vi "host.vi"() -> ()   [LabVIEW 2020]
uses:
  b4957acc-33c7-4f51-b6c8-be02e890b770.vi
  <vilib>/Array/Sort 2D Array - Pop Stack.vi
  <vilib>/Array/Sort 2D Array - Push Stack.vi
  b4957acc-33c7-4f51-b6c8-be02e890b770.vi/269d4b3b-47f5-49e3-8884-44851e4dd9d5.vi
  b4957acc-33c7-4f51-b6c8-be02e890b770.vi/6d99389c-673d-4efb-bf33-19b32bcf4cf8.vi
  <vilib>/FPGAPlugInAG/cRIO-9035/niLvFpga_Open_cRIO-9035.vi
  <vilib>/FPGAPlugInAG/cRIO-9035/niLvFpga_Reset_cRIO-9035.vi
  <vilib>/Utility/error.llb/Error Cluster From Error Code.vi
  <vilib>/rvi/errors/niLvFpgaAdjustHostInterfaceError.vi
  <vilib>/FPGAPlugInAG/cRIO-9035/niLvFpga_Run_cRIO-9035.vi
  <vilib>/FPGAPlugInAG/cRIO-9035/niLvFpga_Close_cRIO-9035.vi
  <vilib>/rvi/interface/nirviOpenFPGA/nirviOpenFPGA.xnode
  FPGA Bitfiles/project_FPGATarget_target_0bYJLxOeBdk.lvbitx
  target.vi
  <vilib>/rvi/interface/nirviMethod/nirviMethod.xnode
  <vilib>/rvi/interface/nirviReadWriteControl/nirviReadWriteControl.xnode
  <vilib>/rvi/interface/nirviCloseFPGA/nirviCloseFPGA.xnode
  <vilib>/Analysis/NI_AALBase.lvlib
  <vilib>/FPGAPlugInAG/cRIO-9035/niLvFpga_StartFifo_cRIO-9035.vi
  <vilib>/rvi/errors/niLvFpgaMergeErrorWithErrorCode.vi
  <vilib>/FPGAPlugInAG/cRIO-9035/niLvFpga_ReadFifo_cRIO-9035.vi
  <vilib>/FPGAPlugInAG/cRIO-9035/niLvFpga_WriteFifo_cRIO-9035.vi
  NiFpgaLv.dll
panel:
  out "LabVIEW sorted array with index 2":sgl[][](array[numeric])
  out "FPGA sorted array with index":sgl[][](array[numeric])
  out "Elements Remaining index":u32
  out "Data":sgl[](array[numeric])
  out "error out":errorcluster
  out "Timed Out? FIFO out IMG":bool
  out "Timed Out? FIFO out REAL":bool
  out "Timed Out? FIFO in REAL":bool
  out "input data":sgl[](graph)
  out "sort time (ms)":dbl
  out "Elements Remaining":u32
  out "Real sorted signal":sgl[](graph)
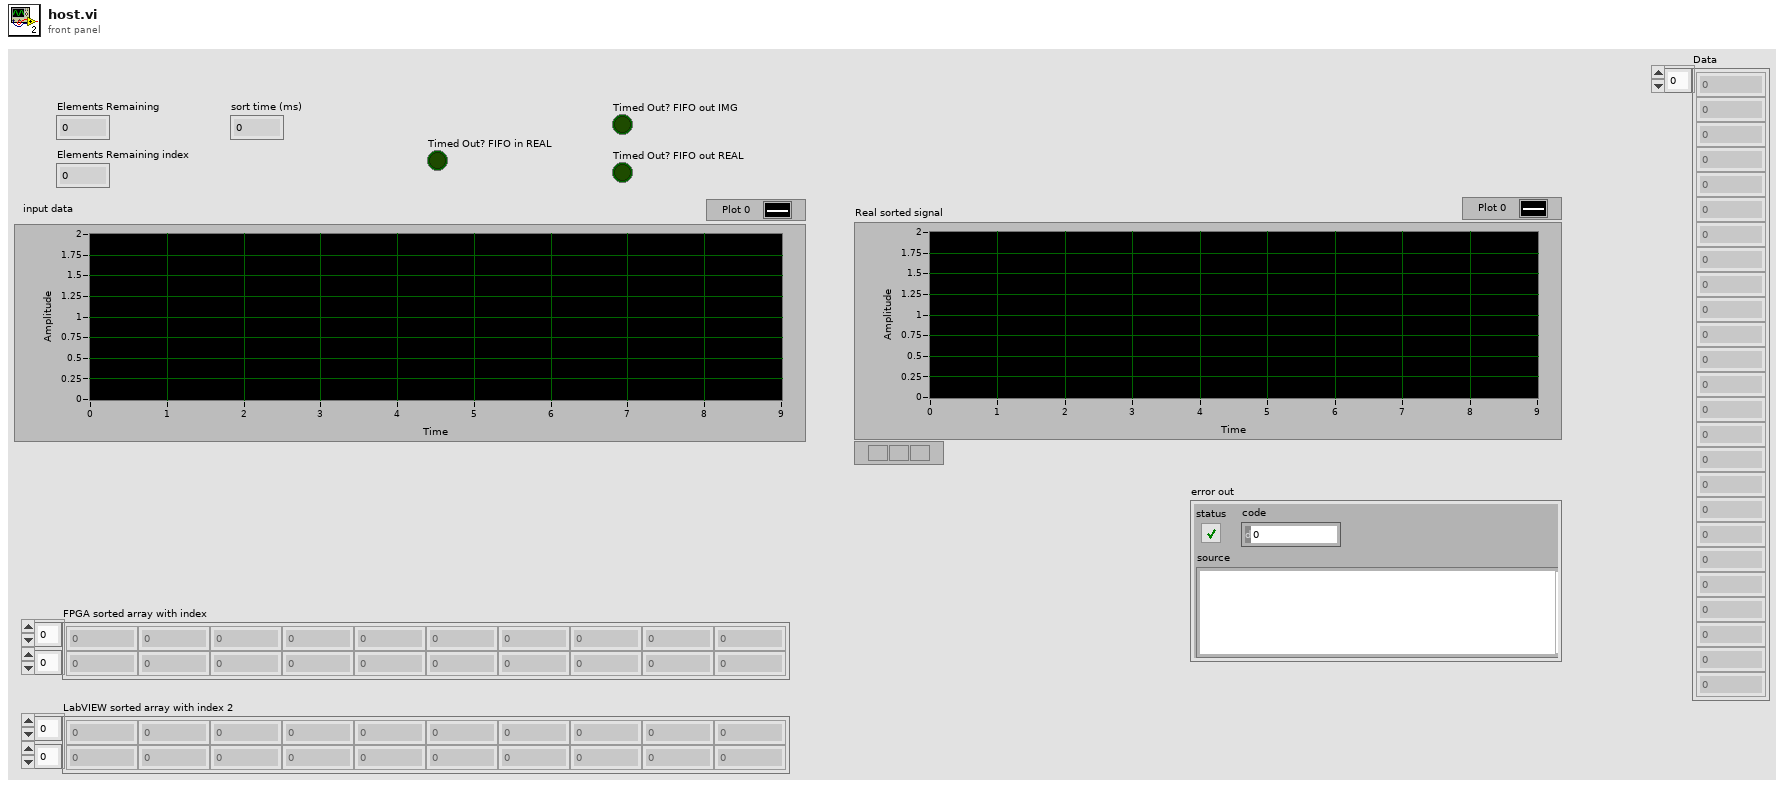
[diagram p1: front panel]
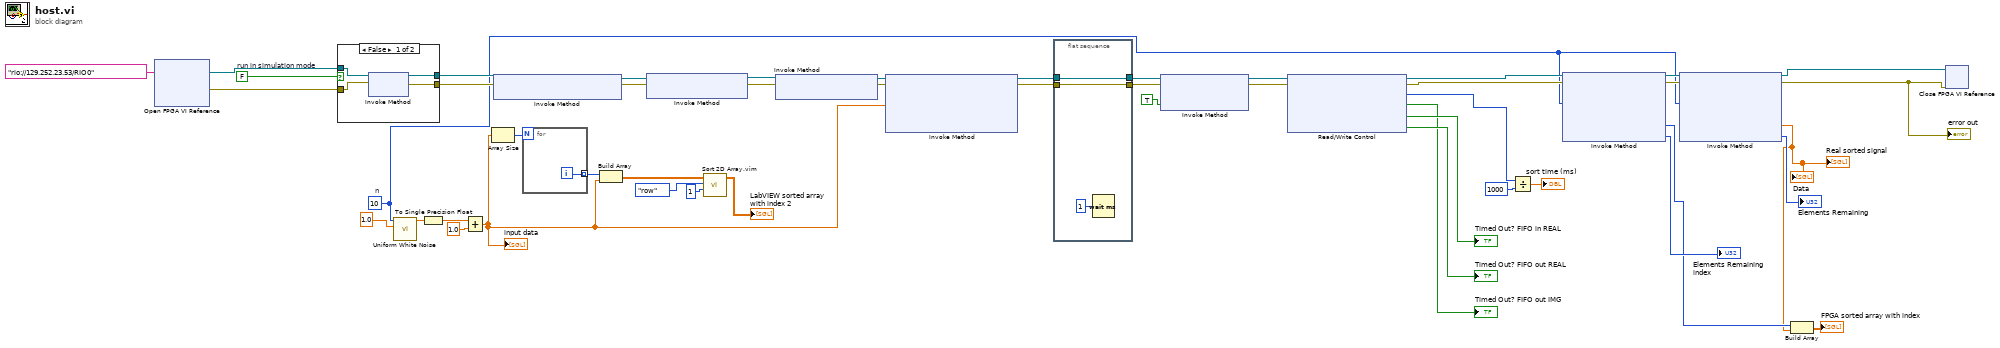
[diagram p0: block diagram]
diagram:
  w15 = FALSE  # run in simulation mode
  w6 = 10  # n
  n1 = xnode "Open FPGA VI Reference"("resource name"=tag "rio://129.252.23.53/RIO0") -> ("FPGA VI Reference Out"=w14:refnum<k20>, "error out"=w13:errorcluster)  [unwired: 1 in]
  n2 = case shown="False" w15 {
    tunnel: w14 -> [w52 w53]
    tunnel: w13 -> [w51 w54]
    tunnel: [w50 w53] -> w12
    tunnel: [w49 w54] -> w11
    frame False {
      n3 = xnode "Invoke Method"("FPGA VI Reference In"=w52, "error in"=w51) -> ("FPGA VI Reference Out"=w50:refnum<k20>, "error out"=w49:errorcluster)
    }
    frame True {
    }
  }
  n4 = call <vilib>:"Uniform White Noise.vi"("amplitude"=1.0, "samples"=w6) -> ("uniform white noise"=w29:dbl[])  [unwired: 8 in, 1 out]
  n5 = To Single Precision Float(number=w29) -> (single precision float=w28:sgl[])
  n6 = Add(x=w28, y=sgl 1.0 ("amplitude")) -> (x+y=w10:sgl[])
  "input data" <- w10
  n7 = Array Size(array=w10) -> (size(s)=w34:i32)
  n8 = xnode "Invoke Method"("FPGA VI Reference In"=w12, "error in"=w11) -> ("FPGA VI Reference Out"=w27:refnum<k20>, "error out"=w26:errorcluster)
  n9 = for {
    N: w34 -> [_]
    tunnel: [w55] -> w33 mode=indexing
    i -> [w55]
  }
  n10 = Build Array(w33, w10) -> (w32:sgl[][])
  n11 = xnode "Invoke Method"("FPGA VI Reference In"=w27, "error in"=w26) -> ("FPGA VI Reference Out"=w20:refnum<k20>, "error out"=w21:errorcluster)
  n12 = call "Sort 2D Array.vim"("index"=1, "dimension to index (column)"=enum16{"column", "row"}."row", "2D array"=w32) -> ("sorted 2D array"=→"LabVIEW sorted array with index 2":sgl[][])  [unwired: 7 in, 1 out]
  n13 = xnode "Invoke Method"("FPGA VI Reference In"=w20, "error in"=w21) -> ("FPGA VI Reference Out"=w25:refnum<k20>, "error out"=w24:errorcluster)
  n14 = xnode "Invoke Method"("FPGA VI Reference In"=w25, "error in"=w24, "Data"=w10) -> ("FPGA VI Reference Out"=w23:refnum<k20>, "error out"=w22:errorcluster)  [unwired: 1 in, 1 out]
  n15 = flat-sequence {
    tunnel: [w57] -> w17
    tunnel: w23 -> [w57]
    tunnel: [w56] -> w16
    tunnel: w22 -> [w56]
    frame #0 {
      n16 = Wait (ms)(milliseconds to wait=u32 1) -> ()  [unwired: 1 out]
    }
  }
  n17 = xnode "Invoke Method"("FPGA VI Reference In"=w17, "error in"=w16, "Wait Until Done (F)"=TRUE) -> ("FPGA VI Reference Out"=w45:refnum<k20>, "error out"=w44:errorcluster)
  n18 = xnode "Read/Write Control"("FPGA VI Reference In"=w45, "error in"=w44) -> ("FPGA VI Reference Out"=w40:refnum<k20>, "error out"=w38:errorcluster, "sort time (us)"=w43:u32, "Timed Out? FIFO out index"=→"Timed Out? FIFO out IMG":bool, "Timed Out? FIFO in REAL"=→"Timed Out? FIFO in REAL":bool, "Timed Out? FIFO out REAL"=→"Timed Out? FIFO out REAL":bool)
  n19 = Divide(x=w43, y=u32 1000) -> (x/y=→"sort time (ms)":dbl)
  n20 = xnode "Invoke Method"("FPGA VI Reference In"=w40, "error in"=w38, "Number of Elements"=w6) -> ("FPGA VI Reference Out"=w39:refnum<k20>, "error out"=w37:errorcluster, "Data"=w4:i32[], "Elements Remaining"=→"Elements Remaining index":u32)  [unwired: 1 in]
  n21 = xnode "Invoke Method"("FPGA VI Reference In"=w39, "error in"=w37, "Number of Elements"=w6) -> ("FPGA VI Reference Out"=w9:refnum<k20>, "error out"=w8:errorcluster, "Data"=w3:sgl[], "Elements Remaining"=→"Elements Remaining":u32)  [unwired: 1 in]
  "Real sorted signal" <- w3
  "error out" <- w8
  "Data" <- w3
  n22 = Build Array(w4, w3) -> (→"FPGA sorted array with index":sgl[][])
  n23 = xnode "Close FPGA VI Reference"("FPGA VI Reference In"=w9, "error in"=w8) -> ()  [unwired: 1 out]
